vi "TCPlogTransaction.vi"(0 "Dashboard Server in":refnum<class "Dashboard Server.lvclass">, 2 "Transaction":string, 5 "error in (no error)":errorcluster) -> (14 "Dashboard Server out":refnum<class "Dashboard Server.lvclass">)   [LabVIEW 2019, in "Dashboard Server.lvclass"]
uses:
  Dashboard Server.lvclass
  Dashboard Server.lvclass/Dashboard Server.ctl
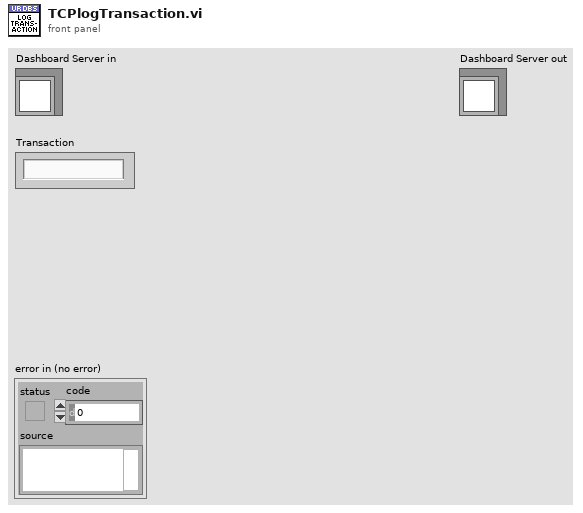
[diagram p1: front panel]
types:
  T1 = enum16{"open", "replace", "create", "open or create", "replace or create", "replace or create with confirmation"}
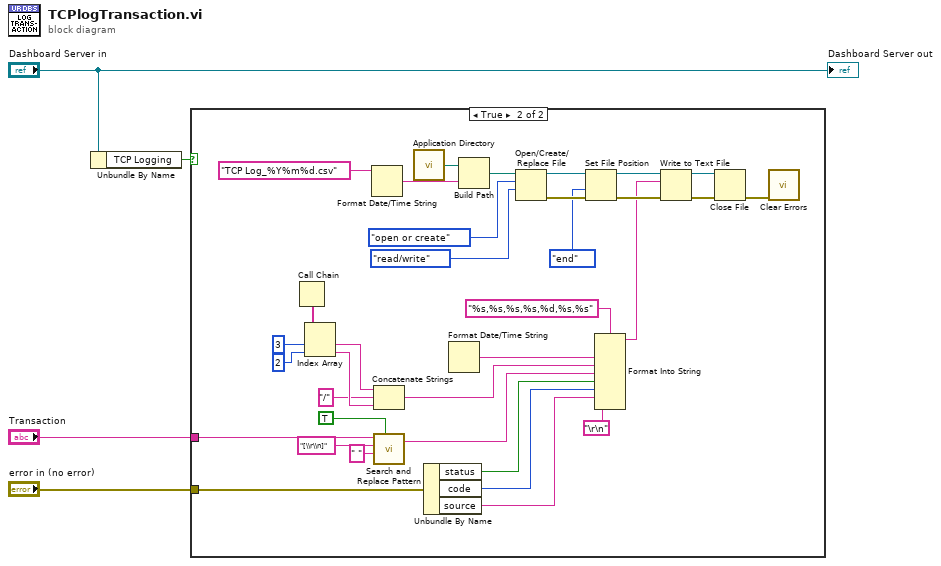
[diagram p0: block diagram]
diagram:
  n1 = Unbundle By Name("Dashboard Server in") -> ("TCP Logging"=w1:bool)
  n2 = case shown="True" w1 {
    tunnel: "Transaction" -> [_ w6]
    tunnel: "error in (no error)" -> [_ w18]
    frame False {
    }
    frame True {
      n3 = Call Chain() -> (call chain=w19:string[])
      n4 = Index Array(array=w19, index #1=3 ("index"), index #2=2 ("index")) -> (element #1=w22:string, element #2=w21:string)
      n5 = Format Date/Time String(time format string (%c)="TCP Log_%Y%m%d.csv") -> (date/time string=w38:string)  [unwired: 2 in]
      n6 = Concatenate Strings(w22, "/" ("string"), w21) -> (w16:string)
      n7 = call <vilib>:"Search and Replace Pattern.vi"("string"=w6, "regular expression (\"\")"="[\\r\\n]" ("regular expression (\"\")"), "replace string (\"\")"=" " ("replace string (\"\")"), "replace all? (F)"=TRUE) -> ("result string"=w5:string)  [unwired: 1 in, 1 out]
      n8 = call <vilib>:"Application Directory.vi"() -> ("Application Directory"=w26:path)
      n9 = Unbundle By Name(w18) -> ("status"=w15:bool, "code"=w14:i32, "source"=w13:string)
      n10 = Format Date/Time String() -> (date/time string=w17:string)  [unwired: 3 in]
      n11 = Build Path(base path=w26, name or relative path=w38) -> (appended path=w37:path)
      n12 = Open/Create/Replace File(file path (use dialog)=w37, operation (0:open)=T1."open or create", access (0:read/write)=enum16{"read/write", "read-only", "write-only"}."read/write") -> (refnum out=w29:refnum<file>, error out=w28:errorcluster)  [unwired: 3 in, 1 out]
      n13 = Set File Position(refnum=w29, from (0:start)=enum16{"start", "end", "current"}."end", error in=w28) -> (refnum out=w33:refnum<file>, error out=w32:errorcluster)  [unwired: 1 in]
      n14 = Format Into String(format string="%s,%s,%s,%s,%d,%s,%s", w17, w16, w5, w15, w14, w13, "\r\n") -> (resulting string=w12:string)  [unwired: 2 in, 1 out]
      n15 = Write to Text File(file (use dialog)=w33, text=w12, error in=w32) -> (refnum out=w31:refnum<file>, error out=w30:errorcluster)  [unwired: 1 in, 1 out]
      n16 = Close File(refnum=w31, error in=w30) -> (error out=w25:errorcluster)  [unwired: 1 out]
      n17 = call <vilib>:"Clear Errors.vi"("error in (no error)"=w25) -> ()  [unwired: 5 in, 2 out]
    }
  }
  "Dashboard Server out" <- "Dashboard Server in"
